vi "ReadthreeLettersPolar.vi"() -> ()   [LabVIEW 2018]
panel:
  out "Array 4":dbl[](array[numeric])
  out "Array 3":dbl[](array[numeric])
  out "third array":dbl[][](array[numeric])
  out "second array":dbl[][](array[numeric])
  out "first":dbl[][](array[numeric])
  in  "Enter initials":string
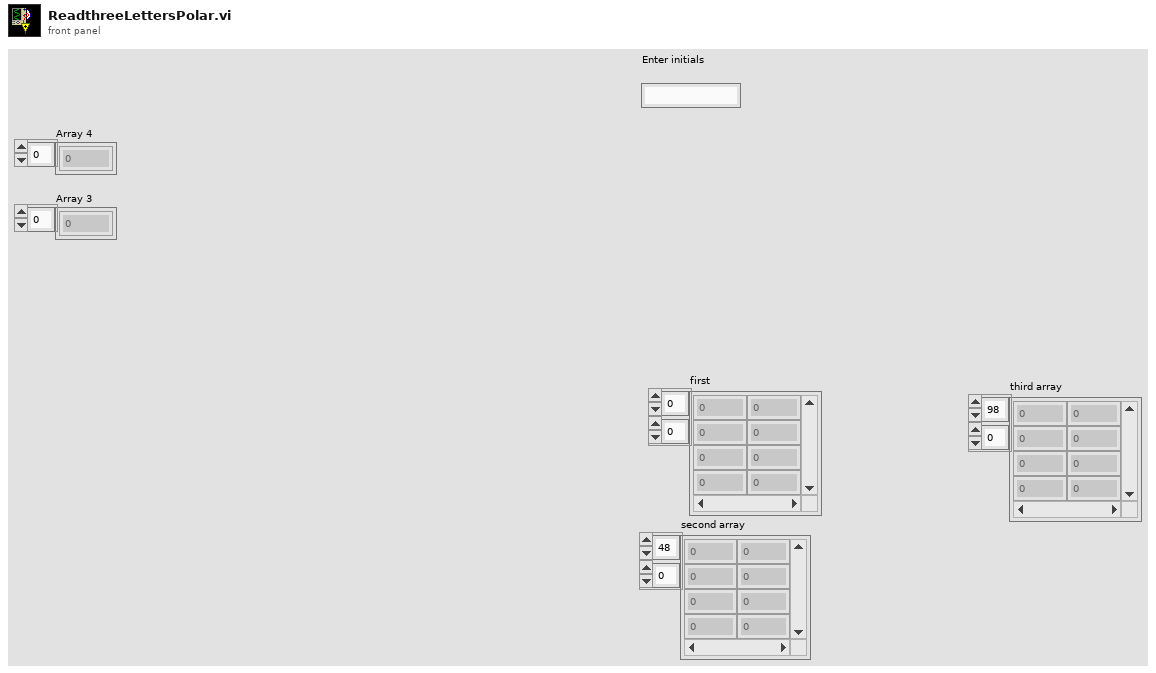
[diagram p1: front panel]
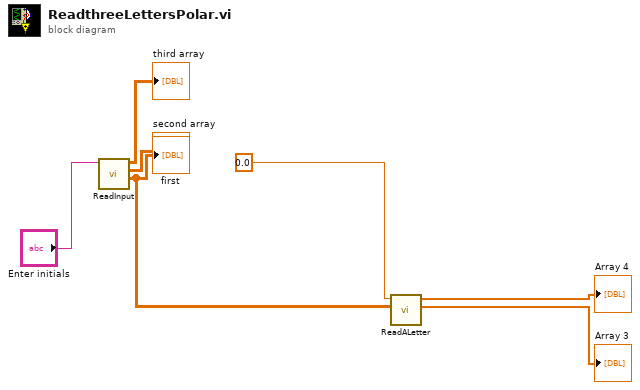
[diagram p0: block diagram]
diagram:
  n1 = call "ReadInput.vi"("Enter initials"="Enter initials") -> ("all rows 3"=w3:dbl[][], "all rows 2"=→"second array":dbl[][], "all rows"=→"third array":dbl[][])  [unwired: 8 in]
  "first" <- w3
  n2 = call "ReadALetter.vi"("all rows 3"=w3, "x"=0.0) -> ("Array 3"=→"Array 3":dbl[], "Array 4"=→"Array 4":dbl[])  [unwired: 8 in]
